vi "Asteroid_object.vi"(7 "Asteroid_states":T1, 8 "error in":errorcluster, 11 "DataIn":variant) -> (0 "error out":errorcluster)   [LabVIEW 2017]
uses:
  Asteroid_states.ctl
  Asteroid_data.ctl
  GameConfig/GameConfig_data.ctl
  ManageMovableObjects/HoldData/DataForColision.ctl
  ManageMovableObjects/HoldData/HoldData_mods.ctl
  ManageMovableObjects/ManRef_mods.ctl
  Display/Display_mods.ctl
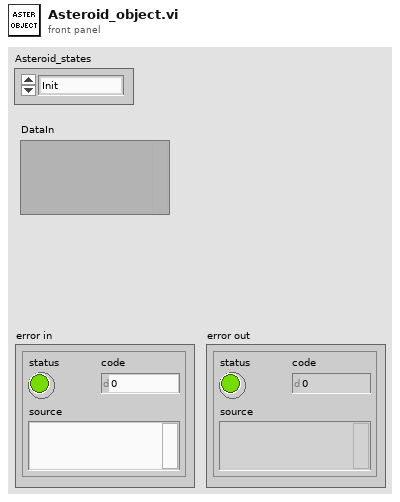
[diagram p1: front panel]
types:
  T1 = typedef "Asteroid_states.ctl" = enum16{"Init", "Move", "Split", "Draw", "Destroy"}
  T2 = typedef "HoldData_mods.ctl" = enum16{"Init", "NewAster", "UpdateAster", "RemoveAster", "GetAsterData", "NewShoot", "UpdateShoot", "RemoveShoot", "GetShootData", "End"}
  T3 = typedef "DataForColision.ctl" = cluster{"X":dbl, "Y":dbl, "Size":dbl, "ID":i32}
  T4 = typedef "Asteroid_data.ctl" = cluster{"Veloc":dbl, "Direction":dbl, "Size":i32, "displayRef":refnum<vi>, "Max X":dbl, "Max Y":dbl, "Xpos":dbl, "Ypos":dbl, "ID":i32, "Config":T5}
  T5 = typedef "GameConfig_data.ctl" = cluster{"SpaceShip":cluster{"Angle":dbl, "SideLenght":dbl, "MaxLinearVeloc":dbl, "MaxAngularVeloc":dbl, "LinearAceleration":dbl, "AngularAceleration":dbl}, "Physics":cluster{"LinearDragFactor":dbl, "AngularDragFactor":dbl}, "Asteroids":cluster{"MaxSize":dbl, "MaxDivisions":i32, "MaxVeloc":dbl, "MinVeloc":dbl, "Fill":bool}, "Environment":cluster{"MaxAsteroids":i32, "TimeIncrement":dbl, "AsterProbCreation":dbl, "LogEnabled":bool}, "Shots":cluster{"MinTimeShots":dbl, "ShotSize":dbl, "ShotSpeed":dbl}}
  T6 = typedef "ManRef_mods.ctl" = enum16{"Init", "NewAster", "MoveAll", "DestroyAster", "NewShoot", "DestroyShot", "CheckColision", "End"}
  T7 = typedef "Display_mods.ctl" = enum16{"Init", "GetBase", "DrawAster", "DrawShip", "DrawShoot", "Clear", "Close"}
  T8 = cluster{"left":i16, "top":i16, "right":i16, "bottom":i16}
  T9 = typedef "LVBoundsTypeDef.ctl" = cluster{"Width":u32, "Height":u32}
  T10 = cluster{"rect":cluster{"left":i16, "top":i16, "right":i16, "bottom":i16}, "Fill":bool}
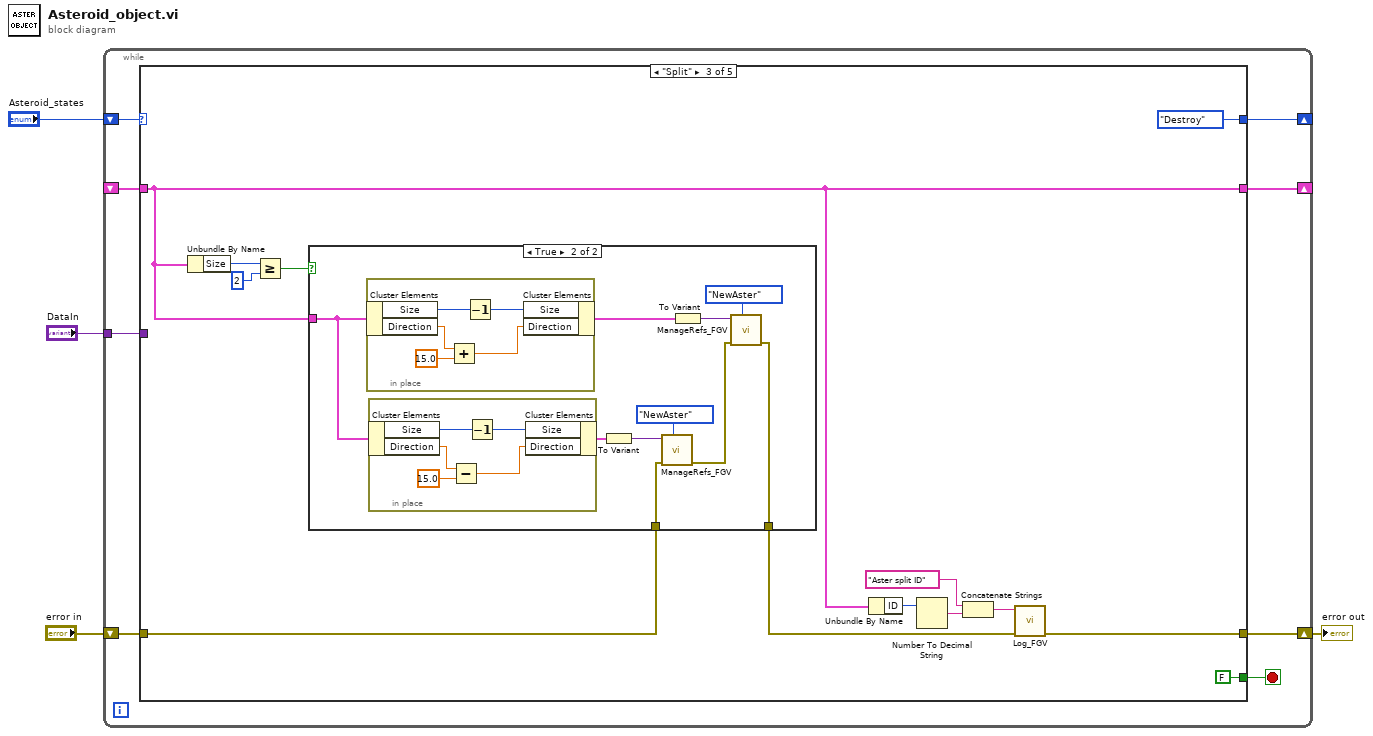
[diagram p0: block diagram]
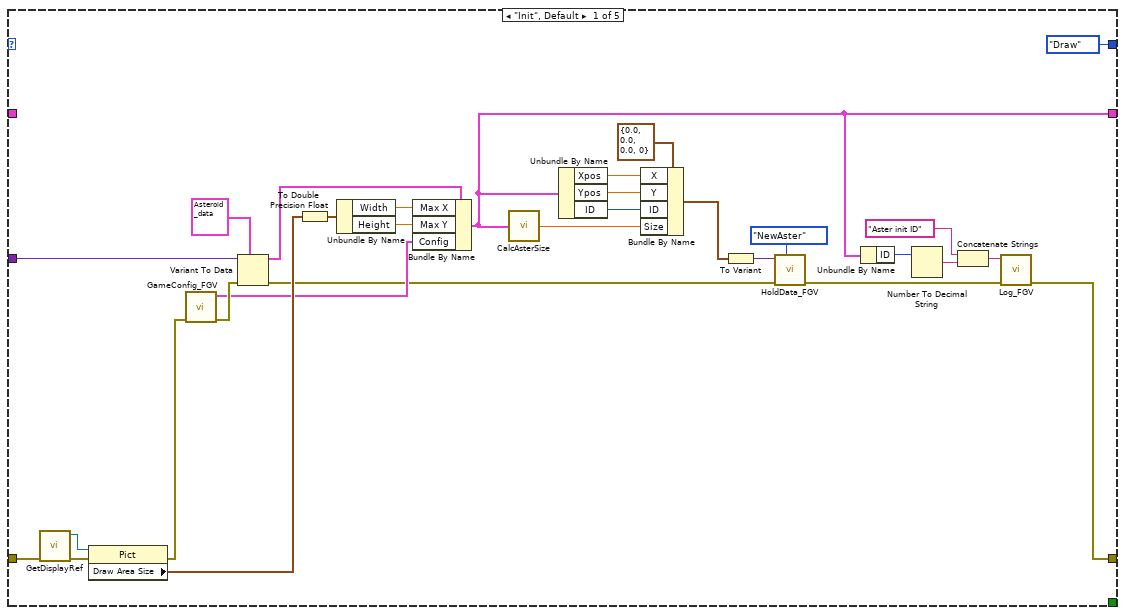
[diagram p2: hidden frame]
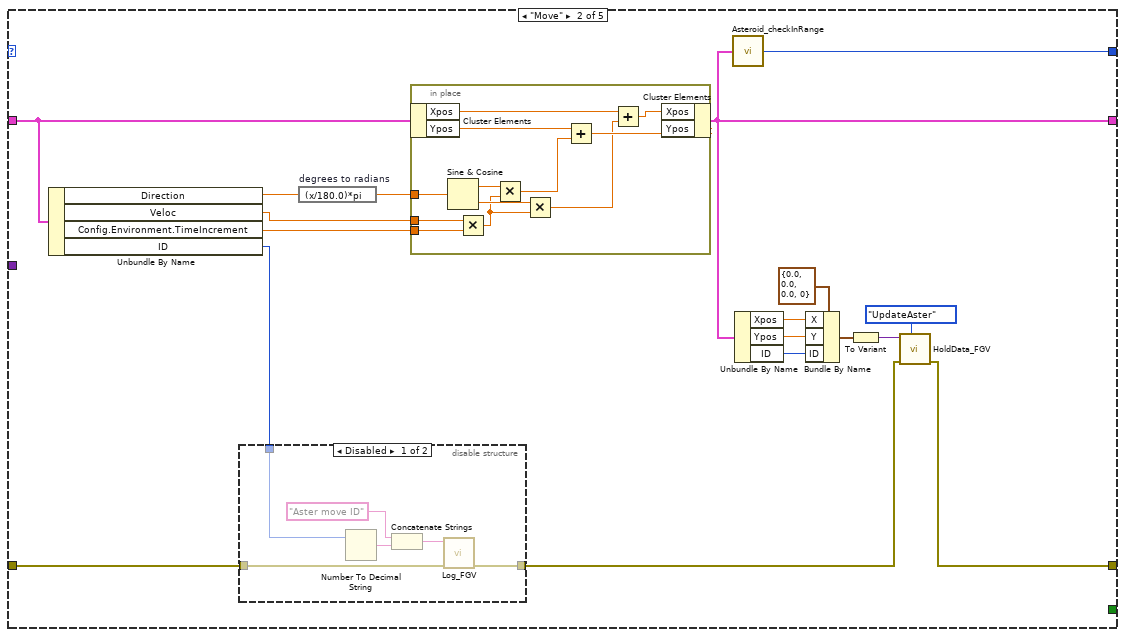
[diagram p3: hidden frame]
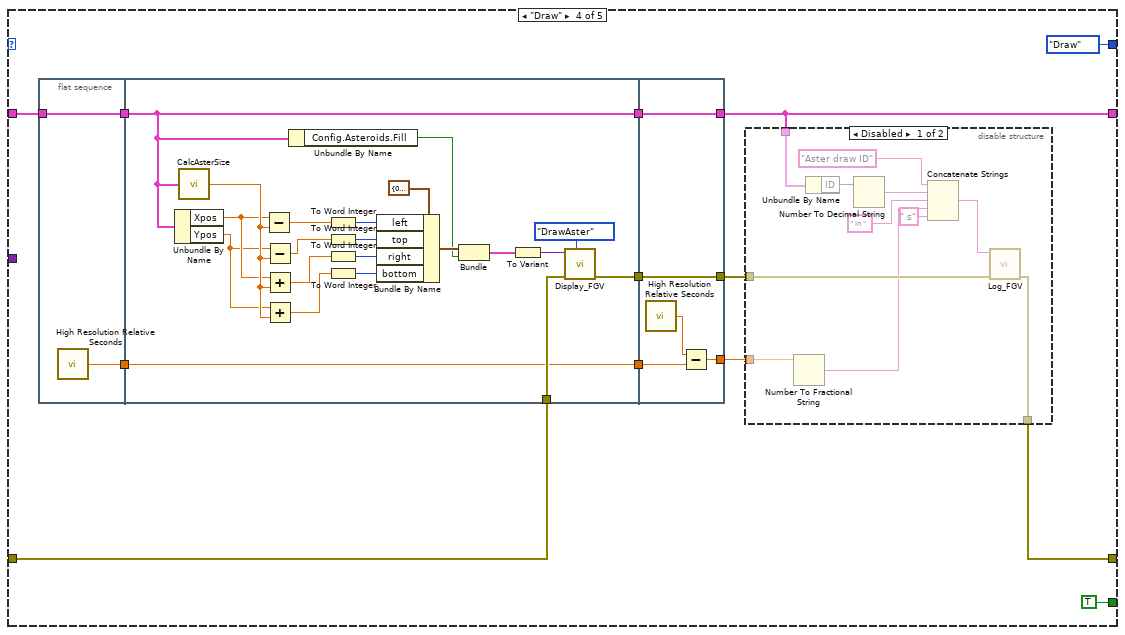
[diagram p6: hidden frame]
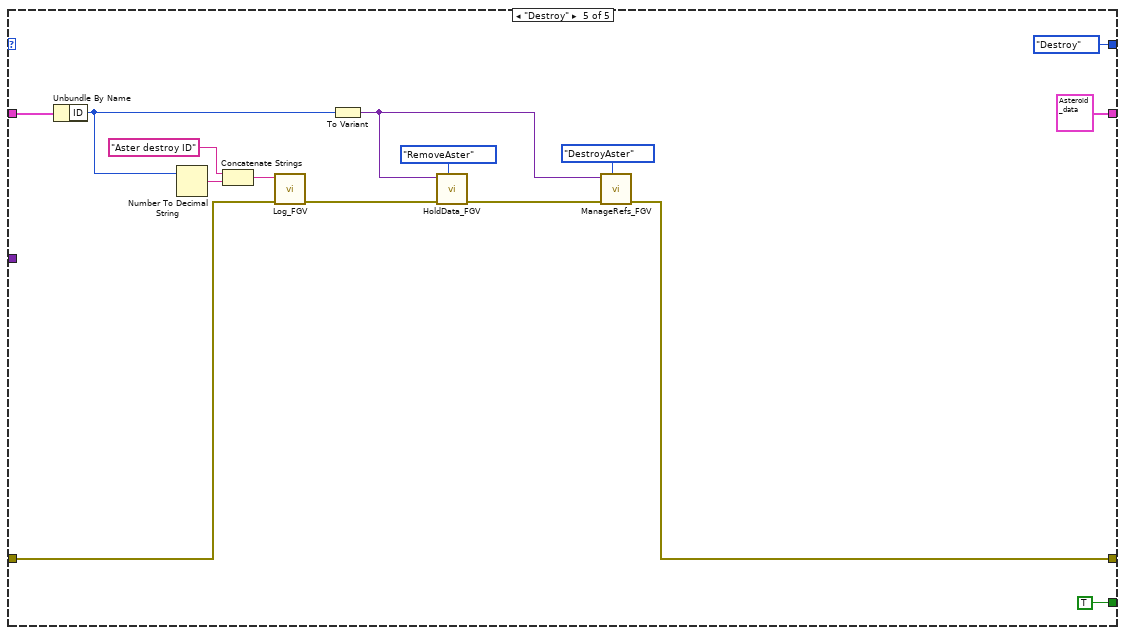
[diagram p8: hidden frame]
diagram:
  n1 = while {
    shift-right: [w10] -> w1
    shift-left: "error in" -> [w11]
    tunnel: "DataIn" -> [w9]
    shift-right: [w8] -> _
    shift-left: _ -> [w7]
    shift-right: [w6] -> _
    shift-left: "Asteroid_states" -> [w12]
    stop <- w5 stop-if-true
    n2 = case shown="\"Split\"" w12 {
      tunnel: w11 -> [w42 w53 w87 w124 w173]
      tunnel: [w29 w43 w82 w122 w168] -> w10
      tunnel: w9 -> [w38 _ _ _ _]
      tunnel: [w18 w45 w81 w120 T4 {"Veloc"=0.0, "Direction"=0.0, "Size"=0, "displayRef"=refnum, "Max X"=0.0, "Max Y"=0.0, "Xpos"=0.0, "Ypos"=0.0, "ID"=0, "Config"={"SpaceShip"={"Angle"=30.0, "SideLenght"=2.0, "MaxLinearVeloc"=10.0, "MaxAngularVeloc"=10.0, "LinearAceleration"=1.0, "AngularAceleration"=1.0}, "Physics"={"LinearDragFactor"=1.0, "AngularDragFactor"=1.0}, "Asteroids"={"MaxSize"=6.0, "MaxDivisions"=3, "MaxVeloc"=8.0, "MinVeloc"=1.0, "Fill"=FALSE}, "Environment"={"MaxAsteroids"=10, "TimeIncrement"=0.1, "AsterProbCreation"=0.1, "LogEnabled"=FALSE}, "Shots"={"MinTimeShots"=10.0, "ShotSize"=0.1, "ShotSpeed"=0.1}}} ("AsteroidData")] -> w8
      tunnel: w7 -> [_ w60 w81 w121 w179]
      tunnel: [Asteroid_states."Draw" ("NextState") w57 Asteroid_states."Destroy" ("Asteroid_states") Asteroid_states."Draw" ("NextState") Asteroid_states."Destroy" ("NextState")] -> w6
      tunnel: [_ _ FALSE TRUE TRUE] -> w5
      frame "Init", Default {
        n3 = call "GetDisplayRef.vi"("error in"=w42) -> ("error out"=w41:errorcluster, "Picture out"=w40:refnum<vi>)  [unwired: 9 in]
        n4 = property class="Pict"(reference=w40, error in=w41) -> (error out=w32:errorcluster, "Draw Area Size"=w39:T9)  [unwired: 1 out]
        n5 = call "GameConfig_FGV.vi"("error in"=w32) -> ("error out"=w31:errorcluster, "Config"=w30:T5)  [unwired: 9 in]
        n6 = Variant To Data(error in=w31, type=T4 {"Veloc"=0.0, "Direction"=0.0, "Size"=0, "displayRef"=refnum, "Max X"=0.0, "Max Y"=0.0, "Xpos"=0.0, "Ypos"=0.0, "ID"=0, "Config"={"SpaceShip"={"Angle"=30.0, "SideLenght"=2.0, "MaxLinearVeloc"=10.0, "MaxAngularVeloc"=10.0, "LinearAceleration"=1.0, "AngularAceleration"=1.0}, "Physics"={"LinearDragFactor"=1.0, "AngularDragFactor"=1.0}, "Asteroids"={"MaxSize"=6.0, "MaxDivisions"=3, "MaxVeloc"=8.0, "MinVeloc"=1.0, "Fill"=FALSE}, "Environment"={"MaxAsteroids"=10, "TimeIncrement"=0.1, "AsterProbCreation"=0.1, "LogEnabled"=FALSE}, "Shots"={"MinTimeShots"=10.0, "ShotSize"=0.1, "ShotSpeed"=0.1}}} ("AsteroidData"), Variant=w38) -> (data=w24:T4, error out=w14:errorcluster)
        n7 = To Double Precision Float(number=w39) -> (double precision float=w36:cluster{"Width":dbl, "Height":dbl})
        n8 = Unbundle By Name(w36) -> ("Width"=w35:dbl, "Height"=w34:dbl)
        n9 = Bundle By Name(cluster=w24, "Max X"=w35, "Max Y"=w34, "Config"=w30) -> (w18:T4)
        n10 = call "CalcAsterSize.vi"("AsteroidData"=w18) -> ("AsteroidSize"=w22:dbl)
        n11 = Unbundle By Name(w18) -> ("Xpos"=w21:dbl, "Ypos"=w20:dbl, "ID"=w19:i32)
        n12 = Bundle By Name(cluster=T3 {"X"=0.0, "Y"=0.0, "Size"=0.0, "ID"=0} ("DataForColision"), "X"=w21, "Y"=w20, "ID"=w19, "Size"=w22) -> (w17:T3)
        n13 = To Variant(anything=w17) -> (Variant=w16:variant)
        n14 = call "HoldData_FGV.vi"("HoldData_mods"=HoldData_mods."NewAster", "error in"=w14, "DataIn"=w16) -> ("error out"=w13:errorcluster)  [unwired: 7 in, 1 out]
        n15 = Unbundle By Name(w18) -> ("ID"=w28:i32)
        n16 = Number To Decimal String(number=w28) -> (decimal integer string=w27:string)  [unwired: 1 in]
        n17 = Concatenate Strings("Aster init ID" ("Log"), w27) -> (w25:string)
        n18 = call "Log_FGV.vi"("error in"=w13, "Log"=w25) -> ("error out"=w29:errorcluster)  [unwired: 9 in]
      }
      frame "Move" {
        n19 = Unbundle By Name(w60) -> ("Direction"=w56:dbl, "Veloc"=w59:dbl, "Config.Environment.TimeIncrement"=w58:dbl, "ID"=w54:i32)
        n20 = disable-structure shown="Disabled" {
          disable-tunnel: w54 -> [w64 _]
          disable-tunnel: w53 -> [w62 w67]
          disable-tunnel: [w61 w67] -> w44
          frame Disabled {
            n21 = Number To Decimal String(number=w64) -> (decimal integer string=w66:string)  [unwired: 1 in]
            n22 = Concatenate Strings("Aster move ID" ("Log"), w66) -> (w63:string)
            n23 = call "Log_FGV.vi"("error in"=w62, "Log"=w63) -> ("error out"=w61:errorcluster)  [unwired: 9 in]
          }
          frame Enabled {
          }
        }
        n24 = expression code="(x/180.0)*pi" "degrees to radians"(w56) -> (w55:dbl)
        n25 = in-place {
          in-place-border: w59 -> [w79]
          in-place-border: w55 -> [w78]
          in-place-border: w58 -> [w68]
          n26 = in-place-cluster #1(w60) -> ("Xpos"=w70:dbl, "Ypos"=w74:dbl)
          n27 = Sine & Cosine(0:w78) -> (1:w75:dbl, 2:w77:dbl)
          n28 = Multiply(x=w79, y=w68) -> (x*y=w76:dbl)
          n29 = Multiply(x=w75, y=w76) -> (x*y=w73:dbl)
          n30 = Multiply(x=w77, y=w76) -> (x*y=w71:dbl)
          n31 = Add(x=w74, y=w73) -> (x+y=w72:dbl)
          n32 = Add(x=w70, y=w71) -> (x+y=w69:dbl)
          n33 = in-place-cluster #1("Xpos"=w69, "Ypos"=w72) -> (w45:T4)
        }
        n34 = call "Asteroid_checkInRange.vi"("AsteroidData"=w45) -> ("NextState"=w57:T1)
        n35 = Unbundle By Name(w45) -> ("Xpos"=w48:dbl, "Ypos"=w49:dbl, "ID"=w50:i32)
        n36 = Bundle By Name(cluster=T3 {"X"=0.0, "Y"=0.0, "Size"=0.0, "ID"=0} ("DataForColision"), "X"=w48, "Y"=w49, "ID"=w50) -> (w51:T3)
        n37 = To Variant(anything=w51) -> (Variant=w52:variant)
        n38 = call "HoldData_FGV.vi"("HoldData_mods"=HoldData_mods."UpdateAster", "error in"=w44, "DataIn"=w52) -> ("error out"=w43:errorcluster)  [unwired: 7 in, 1 out]
      }
      frame "Split" {
        n39 = Unbundle By Name(w81) -> ("Size"=w90:i32)
        n40 = Greater Or Equal?(x=w90, y=2) -> (x >= y?=w88:bool)
        n41 = case shown="True" w88 {
          tunnel: w81 -> [_ w103]
          tunnel: w87 -> [w93 w96]
          tunnel: [w93 w94] -> w83
          frame False {
          }
          frame True {
            n42 = in-place {
              n43 = in-place-cluster #2(w103) -> ("Size"=w113:i32, "Direction"=w111:dbl)
              n44 = Add(x=w111, y=15.0) -> (x+y=w109:dbl)
              n45 = Decrement(x=w113) -> (x-1=w112:i32)
              n46 = in-place-cluster #2("Size"=w112, "Direction"=w109) -> (w101:T4)
            }
            n47 = in-place {
              n48 = in-place-cluster #3(w103) -> ("Size"=w108:i32, "Direction"=w106:dbl)
              n49 = Subtract(x=w106, y=15.0) -> (x-y=w104:dbl)
              n50 = Decrement(x=w108) -> (x-1=w107:i32)
              n51 = in-place-cluster #3("Size"=w107, "Direction"=w104) -> (w97:T4)
            }
            n52 = To Variant(anything=w97) -> (Variant=w99:variant)
            n53 = call "ManageRefs_FGV.vi"("ManRef_mods"=ManRef_mods."NewAster", "error in"=w96, "DataIn"=w99) -> ("error out"=w95:errorcluster)  [unwired: 8 in]
            n54 = To Variant(anything=w101) -> (Variant=w100:variant)
            n55 = call "ManageRefs_FGV.vi"("ManRef_mods"=ManRef_mods."NewAster", "error in"=w95, "DataIn"=w100) -> ("error out"=w94:errorcluster)  [unwired: 8 in]
          }
        }
        n56 = Unbundle By Name(w81) -> ("ID"=w80:i32)
        n57 = Number To Decimal String(number=w80) -> (decimal integer string=w86:string)  [unwired: 1 in]
        n58 = Concatenate Strings("Aster split ID" ("Log"), w86) -> (w85:string)
        n59 = call "Log_FGV.vi"("error in"=w83, "Log"=w85) -> ("error out"=w82:errorcluster)  [unwired: 9 in]
      }
      frame "Draw" {
        n60 = flat-sequence {
          tunnel: w121 -> [w140]
          tunnel: [w140] -> w119
          tunnel: [w139] -> w116
          tunnel: w124 -> [w148]
          tunnel: w119 -> [w142]
          tunnel: [w143] -> w118
          tunnel: [w142] -> w117
          tunnel: w116 -> [w141]
          tunnel: [w141] -> w115
          tunnel: [w165] -> w120
          tunnel: [w166] -> w123
          tunnel: w118 -> [w166]
          tunnel: w117 -> [w165]
          tunnel: w115 -> [w163]
          tunnel: [w162] -> w114
          frame #0 {
            n61 = call <vilib>:"High Resolution Relative Seconds.vi"() -> ("relative seconds"=w139:dbl)
          }
          frame #1 {
            n62 = Unbundle By Name(w142) -> ("Xpos"=w156:dbl, "Ypos"=w155:dbl)
            n63 = call "CalcAsterSize.vi"("AsteroidData"=w142) -> ("AsteroidSize"=w157:dbl)
            n64 = Subtract(x=w156, y=w157) -> (x-y=w160:dbl)
            n65 = Subtract(x=w155, y=w157) -> (x-y=w158:dbl)
            n66 = Add(x=w156, y=w157) -> (x+y=w151:dbl)
            n67 = Add(x=w155, y=w157) -> (x+y=w150:dbl)
            n68 = Unbundle By Name(w142) -> ("Config.Asteroids.Fill"=w146:bool)
            n69 = To Word Integer(number=w160) -> (16bit integer=w159:i16)
            n70 = To Word Integer(number=w158) -> (16bit integer=w154:i16)
            n71 = To Word Integer(number=w151) -> (16bit integer=w153:i16)
            n72 = To Word Integer(number=w150) -> (16bit integer=w152:i16)
            n73 = Bundle By Name(cluster=T8 {"left"=0, "top"=0, "right"=0, "bottom"=0} ("rect"), "left"=w159, "top"=w154, "right"=w153, "bottom"=w152) -> (w147:T8)
            n74 = Bundle("rect"=w147, "Fill"=w146) -> (w145:T10)  [unwired: 1 in]
            n75 = To Variant(anything=w145) -> (Variant=w144:variant)
            n76 = call "Display_FGV.vi"("Display_mods"=Display_mods."DrawAster", "error in"=w148, "variant"=w144) -> ("error out"=w143:errorcluster)  [unwired: 7 in, 1 out]
          }
          frame #2 {
            n77 = call <vilib>:"High Resolution Relative Seconds.vi"() -> ("relative seconds"=w164:dbl)
            n78 = Subtract(x=w164, y=w163) -> (x-y=w162:dbl)
          }
        }
        n79 = disable-structure shown="Disabled" {
          disable-tunnel: w123 -> [w133 w138]
          disable-tunnel: [w132 w138] -> w122
          disable-tunnel: w120 -> [w131 _]
          disable-tunnel: w114 -> [w130 _]
          frame Disabled {
            n80 = Number To Fractional String(number=w130) -> (F-format string=w128:string)  [unwired: 3 in]
            n81 = Unbundle By Name(w131) -> ("ID"=w135:i32)
            n82 = Number To Decimal String(number=w135) -> (decimal integer string=w137:string)  [unwired: 1 in]
            n83 = Concatenate Strings("Aster draw ID" ("Log"), w137, " in " ("string"), w128, " s" ("string")) -> (w136:string)
            n84 = call "Log_FGV.vi"("error in"=w133, "Log"=w136) -> ("error out"=w132:errorcluster)  [unwired: 9 in]
          }
          frame Enabled {
          }
        }
      }
      frame "Destroy" {
        n85 = Unbundle By Name(w179) -> ("ID"=w170:i32)
        n86 = Number To Decimal String(number=w170) -> (decimal integer string=w176:string)  [unwired: 1 in]
        n87 = Concatenate Strings("Aster destroy ID" ("Log"), w176) -> (w175:string)
        n88 = call "Log_FGV.vi"("error in"=w173, "Log"=w175) -> ("error out"=w171:errorcluster)  [unwired: 9 in]
        n89 = To Variant(anything=w170) -> (Variant=w167:variant)
        n90 = call "HoldData_FGV.vi"("HoldData_mods"=HoldData_mods."RemoveAster", "error in"=w171, "DataIn"=w167) -> ("error out"=w169:errorcluster)  [unwired: 7 in, 1 out]
        n91 = call "ManageRefs_FGV.vi"("ManRef_mods"=ManRef_mods."DestroyAster", "error in"=w169, "DataIn"=w167) -> ("error out"=w168:errorcluster)  [unwired: 8 in]
      }
    }
  }
  "error out" <- w1
